vi "Stop Logging.vi"() -> (0 "error out":errorcluster)   [LabVIEW 2020]
doc: "Stops the logging."
uses:
  sub VIs/Globals.vi
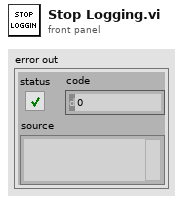
[diagram p1: front panel]
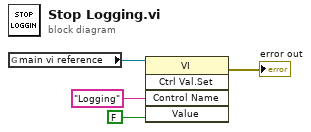
[diagram p0: block diagram]
diagram:
  n1 = global read "Globals.vi" "main vi reference"() -> (w4:refnum<vi>)
  n2 = invoke class="VI" method="Ctrl Val.Set"(reference=w4, "Control Name"="Logging", "Value"=FALSE) -> (error out=→"error out":errorcluster)  [unwired: 2 in, 4 out]
